vi "MB Registers Manager.vi"(6 "Bits In":bool[](array[boolean]), 7 "Table":T2(ring), 8 "error in (no error)":errorcluster, 9 "Words In":u16[](array[numeric]), 10 "Length":u16, 11 "Start Address":u16) -> (0 "error out":errorcluster)   [LabVIEW 2019, in "NI_modbus_upd.lvlib"]
uses:
  NI_modbus_upd.lvlib
panel:
  in  "Data Reference":T1
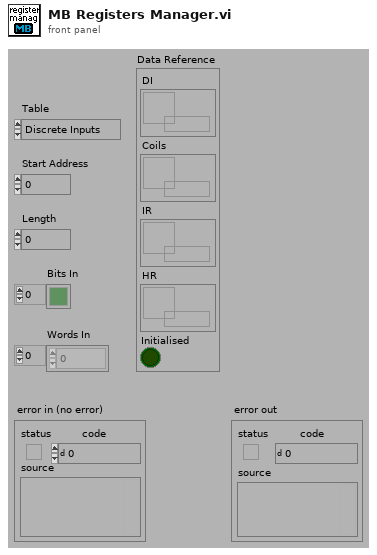
[diagram p1: front panel]
types:
  T1 = cluster{"DI":refnum<data-value>, "Coils":refnum<data-value>, "IR":refnum<data-value>, "HR":refnum<data-value>, "Initialised":bool}
  T2 = enum16{"Discrete Inputs", "Coils", "Input Registers", "Holding Registers"}
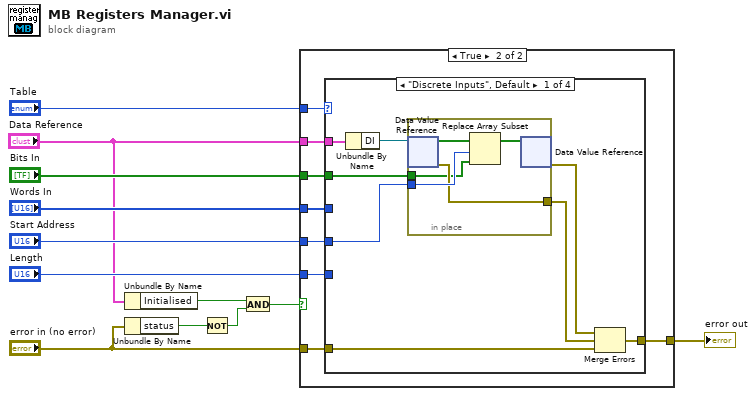
[diagram p0: block diagram]
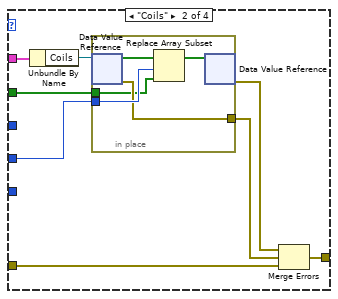
[diagram p3: hidden frame]
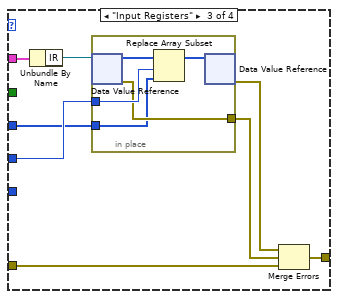
[diagram p4: hidden frame]
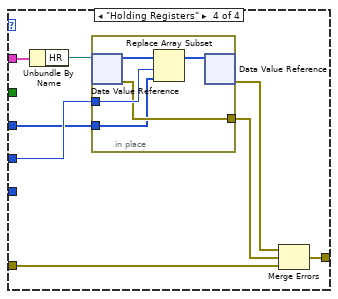
[diagram p5: hidden frame]
diagram:
  n1 = Unbundle By Name("Data Reference") -> ("Initialised"=w3:bool)
  n2 = Unbundle By Name("error in (no error)") -> ("status"=w5:bool)
  n3 = Not(x=w5) -> (.not. x?=w4:bool)
  n4 = And(x=w3, y=w4) -> (x .and. y?=w6:bool)
  n5 = case shown="True" w6 {
    tunnel: [w13 w17] -> w12
    tunnel: "Length" -> [_ w21]
    tunnel: "Start Address" -> [_ w20]
    tunnel: "Bits In" -> [_ w15]
    tunnel: "Words In" -> [_ w14]
    tunnel: "Table" -> [_ w16]
    tunnel: "Data Reference" -> [_ w19]
    tunnel: "error in (no error)" -> [w13 w18]
    frame False {
    }
    frame True {
      n6 = case shown="\"Discrete Inputs\", Default" w16 {
        tunnel: w21 -> [_ _ _ _]
        tunnel: w20 -> [w29 w42 w55 w68]
        tunnel: w19 -> [w28 w41 w54 w67]
        tunnel: w18 -> [w27 w40 w53 w66]
        tunnel: [w24 w37 w50 w63] -> w17
        tunnel: w15 -> [w22 w35 _ _]
        tunnel: w14 -> [_ _ w48 w61]
        frame "Discrete Inputs", Default {
          n7 = Unbundle By Name(w28) -> ("DI"=w23:refnum<data-value>)
          n8 = in-place {
            in-place-border: w29 -> [w34]
            in-place-border: [w33] -> w25
            in-place-border: w22 -> [w30]
            n9 = in-place-dvr #1(w23) -> (w32:bool[], w33:errorcluster)
            n10 = Replace Array Subset(array=w32, new element=w30, index=w34) -> (w31:bool[])
            n11 = in-place-dvr #1(w31) -> (w26:errorcluster)  [unwired: 1 out]
          }
          n12 = Merge Errors(w26, w25, w27) -> (w24:errorcluster)
        }
        frame "Coils" {
          n13 = Unbundle By Name(w41) -> ("Coils"=w36:refnum<data-value>)
          n14 = in-place {
            in-place-border: w42 -> [w47]
            in-place-border: [w46] -> w38
            in-place-border: w35 -> [w43]
            n15 = in-place-dvr #2(w36) -> (w45:bool[], w46:errorcluster)
            n16 = Replace Array Subset(array=w45, new element=w43, index=w47) -> (w44:bool[])
            n17 = in-place-dvr #2(w44) -> (w39:errorcluster)  [unwired: 1 out]
          }
          n18 = Merge Errors(w39, w38, w40) -> (w37:errorcluster)
        }
        frame "Input Registers" {
          n19 = Unbundle By Name(w54) -> ("IR"=w49:refnum<data-value>)
          n20 = in-place {
            in-place-border: w55 -> [w60]
            in-place-border: [w59] -> w51
            in-place-border: w48 -> [w56]
            n21 = in-place-dvr #3(w49) -> (w58:u16[], w59:errorcluster)
            n22 = Replace Array Subset(array=w58, new element=w56, index=w60) -> (w57:u16[])
            n23 = in-place-dvr #3(w57) -> (w52:errorcluster)  [unwired: 1 out]
          }
          n24 = Merge Errors(w52, w51, w53) -> (w50:errorcluster)
        }
        frame "Holding Registers" {
          n25 = Unbundle By Name(w67) -> ("HR"=w62:refnum<data-value>)
          n26 = in-place {
            in-place-border: w68 -> [w73]
            in-place-border: [w72] -> w64
            in-place-border: w61 -> [w69]
            n27 = in-place-dvr #4(w62) -> (w71:u16[], w72:errorcluster)
            n28 = Replace Array Subset(array=w71, new element=w69, index=w73) -> (w70:u16[])
            n29 = in-place-dvr #4(w70) -> (w65:errorcluster)  [unwired: 1 out]
          }
          n30 = Merge Errors(w65, w64, w66) -> (w63:errorcluster)
        }
      }
    }
  }
  "error out" <- w12
